vi "Trial.vi"(2 "error in (no error)":errorcluster, 3 "DDA":bool=TRUE) -> (0 "error out":errorcluster)   [LabVIEW 2017]
uses:
  Control/RPY.ctl
  Control/Parameter Theta.ctl
  Control/State.ctl
  <vilib>/Analysis/_algsub.llb/Real Vector Norm.vi
  <vilib>/Analysis/baseanly.llb/A x Vector.vi
  <vilib>/Analysis/baseanly.llb/Outer Product.vi
  <vilib>/Analysis/baseanly.llb/Real Outer Product.vi
  <vilib>/robotics/Kinematics/Create Lie Group Matrix.vi
  Global.vi
  <vilib>/Analysis/7linalg.llb/Create Special Matrix.vi
  <vilib>/Analysis/7linalg.llb/Create Special Real Matrix.vi
  <vilib>/Analysis/Matrix/Numeric/Multiply/Multiply.vi
  <vilib>/Analysis/Matrix/Numeric/Multiply/Multiply - RM,R.vi
  <vilib>/Analysis/Matrix/Numeric/Multiply/Multiply - R,RM.vi
  <vilib>/Analysis/Matrix/Numeric/Add/Add.vi
  <vilib>/Analysis/Matrix/Numeric/Add/Add - RM,RM.vi
  <vilib>/Analysis/NI_AALPro.lvlib
  <vilib>/robotics/Kinematics/NI_Kinematics.lvlib
  <vilib>/Analysis/NI_AALBase.lvlib
panel:
  out "Trial":i32
  in  "Time Target (s)":dbl=10.0
  in  "epsilon":dbl=0.1
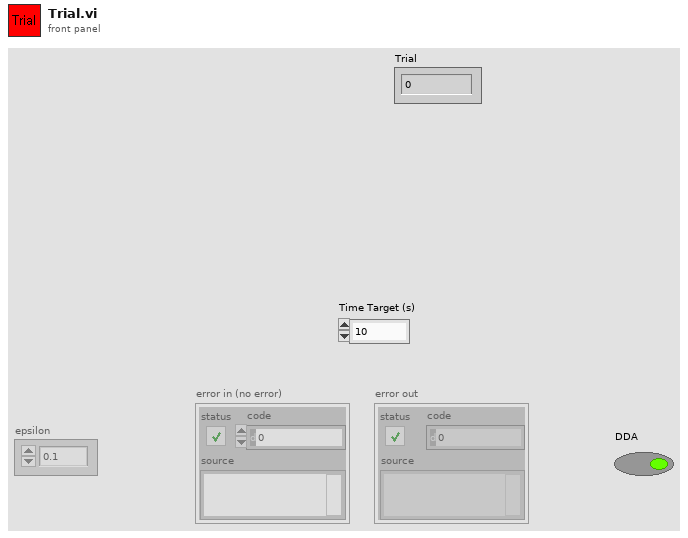
[diagram p1: front panel]
types:
  T1 = typedef "Parameter Theta.ctl" = cluster{"thI":dbl[][], "thD":dbl[][], "thR":dbl[][]}
  T2 = typedef "RPY.ctl" = cluster{"roll":dbl, "pitch":dbl, "yaw":dbl}
  T3 = typedef "State.ctl" = cluster{"Inertia (Kg)":dbl, "Damping (N*s/m)":dbl, "RoM (deg)":dbl}
  T4 = typedef "NI_Matrix.lvlib/RealMatrix.ctl" = dbl[][]
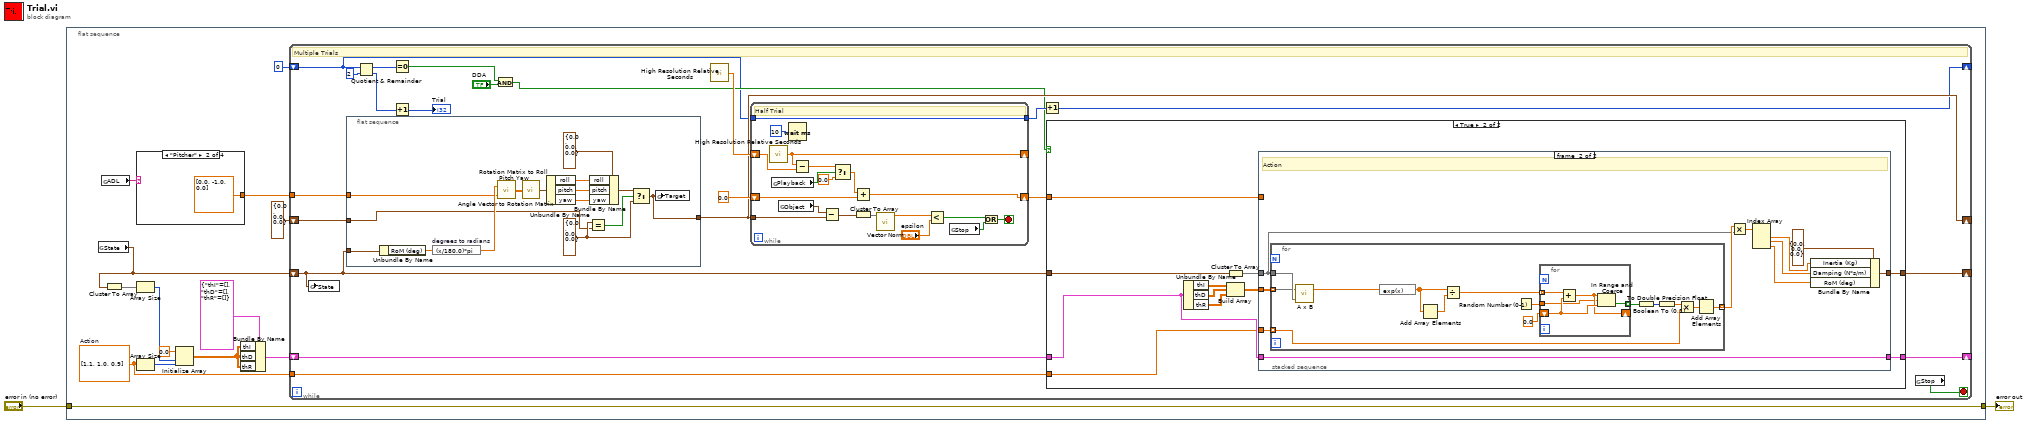
[diagram p0: block diagram]
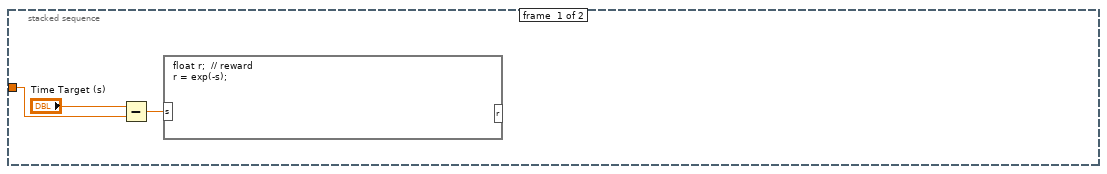
[diagram p3: hidden frame]
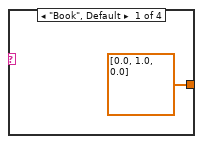
[diagram p4: hidden frame]
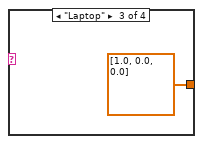
[diagram p5: hidden frame]
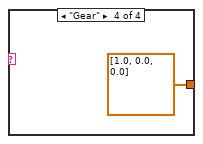
[diagram p6: hidden frame]
diagram:
  n1 = flat-sequence {
    tunnel: [w15] -> w2
    tunnel: "error in (no error)" -> [w15]
    frame #0 {
      w4 = dbl[] [1.1, 1.0, 0.9]  # Action
      n2 = global read "Global.vi" "State"() -> (w3:T3)
      n3 = global read "Global.vi" "ADL"() -> (w16:string)
      n4 = Cluster To Array(cluster=w3) -> (array=w13:dbl[])
      n5 = case shown="\"Pitcher\"" w16 {
        tunnel: [dbl[] [0.0, 1.0, 0.0] dbl[] [0.0, -1.0, 0.0] dbl[] [1.0, 0.0, 0.0] dbl[] [1.0, 0.0, 0.0]] -> w9
        frame "Book", Default {
        }
        frame "Pitcher" {
        }
        frame "Laptop" {
        }
        frame "Gear" {
        }
      }
      n6 = Array Size(array=w13) -> (size(s)=w11:i32)
      n7 = Array Size(array=w4) -> (size(s)=w10:i32)
      n8 = Initialize Array(0.0 ("element"), w11, w10) -> (w6:dbl[][])
      n9 = Bundle By Name(cluster=T1 {"thI"=[], "thD"=[], "thR"=[]} ("Parameter Theta"), "thI"=w6, "thD"=w6, "thR"=w6) -> (w5:T1)
      n10 = while {
        shift-right: [w25] -> _
        shift-left: 0 ("Trial") -> [w19]
        tunnel: w9 -> [w35]
        shift-right: [w34] -> _
        shift-left: w3 -> [w26]
        shift-right: [w32] -> _
        shift-left: T2 {"roll"=0.0, "pitch"=0.0, "yaw"=0.0} ("Target") -> [w31]
        shift-right: [w30] -> _
        shift-left: w5 -> [w29]
        tunnel: w4 -> [w28]
        stop <- w33 stop-if-true
        # "Multiple Trials"
        n11 = global write "Global.vi" "State"(w26) -> ()
        n12 = flat-sequence {
          tunnel: w35 -> [w45]
          tunnel: w26 -> [w44]
          tunnel: [w40] -> w32
          tunnel: w31 -> [w39]
          frame #0 {
            w41 = T2 {"roll"=0.0, "pitch"=0.0, "yaw"=0.0} ("Target")
            n13 = Unbundle By Name(w44) -> ("RoM (deg)"=w46:dbl)
            n14 = expression code="(x/180.0)*pi" "degrees to radians"(w46) -> (w47:dbl)
            n15 = call <vilib>:"Angle Vector to Rotation Matrix.vi"("vector"=w45, "angle"=w47) -> ("rotation matrix"=w48:T4)
            n16 = call <vilib>:"Rotation Matrix to Roll Pitch Yaw.vi"("rotation matrix"=w48) -> ("angles"=w49:cluster{"roll":dbl, "pitch":dbl, "yaw":dbl})
            n17 = Unbundle By Name(w49) -> ("roll"=w50:dbl, "pitch"=w51:dbl, "yaw"=w52:dbl)
            n18 = Equal?(x=w41, y=w39) -> (x = y?=w53:bool)
            n19 = Bundle By Name(cluster=T2 {"roll"=0.0, "pitch"=0.0, "yaw"=0.0} ("Target"), "roll"=w50, "pitch"=w51, "yaw"=w52) -> (w42:T2)
            n20 = Select(t=w42, s=w53, f=w41) -> (s? t:f=w40:T2)
            n21 = global write "Global.vi" "Target"(w40) -> ()
          }
        }
        n22 = Quotient & Remainder(x=w19, y=2) -> (x-y*floor(x/y)=w23:i32, floor(x/y)=w18:i32)
        n23 = Equal To 0?(x=w23) -> (x = 0?=w22:bool)
        n24 = Increment(x=w18) -> (x+1=→"Trial":i32)
        n25 = And(x=w22, y="DDA") -> (x .and. y?=w20:bool)
        n26 = call <vilib>:"High Resolution Relative Seconds.vi"() -> ("relative seconds"=w38:dbl)
        n27 = while {
          tunnel: w32 -> [w113]
          shift-right: [w107] -> _
          shift-left: w38 -> [w108]
          shift-right: [w101] -> w27
          shift-left: 0.0 -> [w106]
          tunnel: [w100] -> w36
          tunnel: w19 -> [w100]
          stop <- w109 stop-if-true
          # "Half Trial"
          n28 = call <vilib>:"High Resolution Relative Seconds.vi"() -> ("relative seconds"=w107:dbl)
          n29 = global read "Global.vi" "Playback"() -> (w105:bool)
          n30 = global read "Global.vi" "Object"() -> (w116:T2)
          n31 = Wait (ms)(milliseconds to wait=u32 10) -> ()  [unwired: 1 out]
          n32 = Subtract(x=w107, y=w108) -> (x-y=w104:dbl)
          n33 = Subtract(x=w116, y=w113) -> (x-y=w117:T2)
          n34 = Select(t=w104, s=w105, f=0.0) -> (s? t:f=w103:dbl)
          n35 = Add(x=w103, y=w106) -> (x+y=w101:dbl)
          n36 = Cluster To Array(cluster=w117) -> (array=w118:dbl[])
          n37 = call-poly <vilib>:"Vector Norm.vi"("Input Vector"=w118) -> ("norm"=w115:dbl)  [unwired: 9 in, 1 out]
          n38 = Less?(x=w115, y="epsilon") -> (x < y?=w112:bool)
          n39 = global read "Global.vi" "Stop"() -> (w111:bool)
          n40 = Or(x=w112, y=w111) -> (x .or. y?=w109:bool)
        }
        n41 = Increment(x=w36) -> (x+1=w25:i32)
        n42 = case shown="True" w20 {
          tunnel: [w55 w65] -> w34
          tunnel: w26 -> [w55 w63]
          tunnel: [w54 w66] -> w30
          tunnel: w29 -> [w54 w62]
          tunnel: w28 -> [_ w57]
          tunnel: w27 -> [_ w56]
          frame False {
          }
          frame True {
            n43 = Unbundle By Name(w62) -> ("thI"=w61:dbl[][], "thD"=w60:dbl[][], "thR"=w59:dbl[][])
            n44 = Build Array(w61, w60, w59) -> (w58:dbl[][][])
            n45 = Cluster To Array(cluster=w63) -> (array=w64:dbl[])
            n46 = stacked-sequence {
              tunnel: [_ w80] -> w66
              tunnel: w62 -> [_ w80]
              tunnel: [_ w73] -> w65
              tunnel: w64 -> [_ w76]
              tunnel: w58 -> [_ w79]
              tunnel: w57 -> [_ w78]
              tunnel: w56 -> [w68 _]
              frame #0 {
                n47 = Subtract(x="Time Target (s)", y=w68) -> (x-y=w67:dbl)
                n48 = formula code="float r;  // reward\nr = exp(-s);"("s"=w67) -> ()  [unwired: 1 out]
              }
              frame #1 {
                # "Action"
                n49 = for {
                  tunnel: w76 -> [w90]
                  tunnel: w79 -> [w89] mode=indexing
                  tunnel: w78 -> [w85] mode=indexing
                  tunnel: [w81] -> w77 mode=indexing
                  n50 = call-poly <vilib>:"A x B.vi"("Vector"=w90, "A"=w89) -> ("A x Vector"=w94:dbl[])  [unwired: 1 out]
                  n51 = expression code="exp(x)"(w94) -> (w93:dbl[])
                  n52 = Add Array Elements(numeric array=w93) -> (sum=w92:dbl)
                  n53 = Divide(x=w93, y=w92) -> (x/y=w88:dbl[])
                  n54 = Random Number (0-1)() -> (number: 0 to 1=w87:dbl)
                  n55 = for {
                    shift-right: [w97] -> _
                    shift-left: 0.0 -> [w99]
                    tunnel: w88 -> [w98] mode=indexing
                    tunnel: w87 -> [w96]
                    tunnel: [w95] -> w86 mode=indexing
                    n56 = Add(x=w98, y=w99) -> (x+y=w97:dbl)
                    n57 = In Range and Coerce(upper limit=w97, x=w96, lower limit=w99) -> (In Range?=w95:bool)  [unwired: 1 out]
                  }
                  n58 = Boolean To (0,1)(Boolean=w86) -> (0, 1=w84:i16[])
                  n59 = To Double Precision Float(number=w84) -> (double precision float=w83:dbl[])
                  n60 = Multiply(x=w83, y=w85) -> (x*y=w82:dbl[])
                  n61 = Add Array Elements(numeric array=w82) -> (sum=w81:dbl)
                }
                n62 = Multiply(x=w77, y=w76) -> (x*y=w74:dbl[])
                n63 = Index Array(array=w74) -> (element #1=w72:dbl, element #2=w71:dbl, element #3=w70:dbl)  [unwired: 3 in]
                n64 = Bundle By Name(cluster=T3 {"Inertia (Kg)"=0.0, "Damping (N*s/m)"=0.0, "RoM (deg)"=0.0} ("State"), "Inertia (Kg)"=w72, "Damping (N*s/m)"=w71, "RoM (deg)"=w70) -> (w73:T3)
              }
            }
          }
        }
        n65 = global read "Global.vi" "Stop"() -> (w33:bool)
      }
    }
  }
  "error out" <- w2
